vi "Start Sync.vi"(8 "error in (no error)":errorcluster, 11 "gRPC Server in":refnum<class "Query Server.lvclass">) -> (0 "error out":errorcluster, 3 "gRPC Server out":refnum<class "Query Server.lvclass">)   [LabVIEW 2019, in "Query Server.lvlib" / "Query Server.lvclass"]
uses:
  Query Server.lvclass
  gRPC lvSupport/Server API/typeDefs/grpcId.ctl
  Query Server.lvclass/Query Server.ctl
  RPC Messages/ServerEvent/ServerEvent_Data.ctl
  RPC Messages/QueryResponse/QueryResponse_Data.ctl
  RPC Messages/InvokeResponse/InvokeResponse_Data.ctl
  gRPC lvSupport/gprc-lvsupport.lvlib
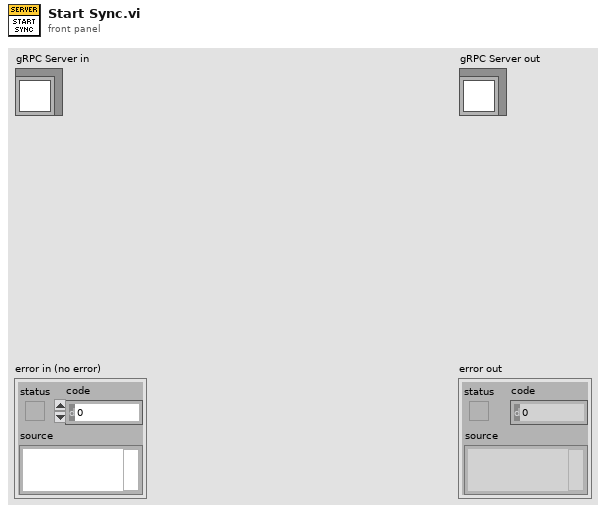
[diagram p1: front panel]
types:
  T1 = typedef "Query Server.lvlib/gprc-lvsupport.lvlib/grpcId.ctl" = u64
  T2 = typedef "Query Server.lvlib/Query Server.lvclass/ServerEvent_Data.ctl" = cluster{"eventData":string, "serverId":i32, "status":i32}
  T3 = typedef "Query Server.lvlib/Query Server.lvclass/QueryResponse_Data.ctl" = cluster{"message":string, "status":i32}
  T4 = typedef "Query Server.lvlib/Query Server.lvclass/InvokeResponse_Data.ctl" = cluster{"status":i32}
  T5 = typedef "Query Server.lvlib/Query Server.lvclass/Server gRPC UEs.ctl" = cluster{"Invoke gRPC UE":refnum<user-event>, "Query gRPC UE":refnum<user-event>, "Register gRPC UE":refnum<user-event>}
  T6 = typedef "Query Server.lvlib/Query Server.lvclass/RegistrationRequest_Data.ctl" = cluster{"eventName":string}
  T7 = typedef "Query Server.lvlib/Query Server.lvclass/QueryRequest_Data.ctl" = cluster{"query":string}
  T8 = typedef "Query Server.lvlib/Query Server.lvclass/InvokeRequest_Data.ctl" = cluster{"command":string, "parameter":string}
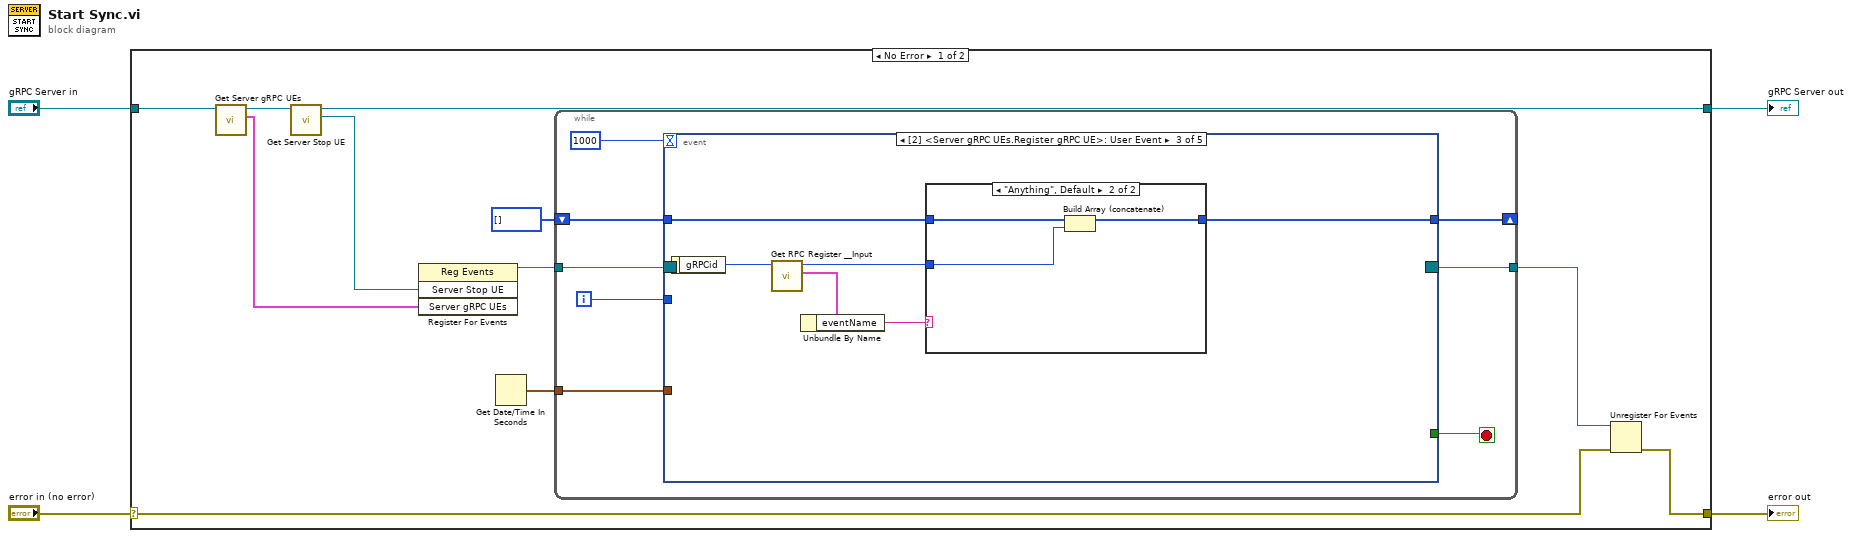
[diagram p0: block diagram]
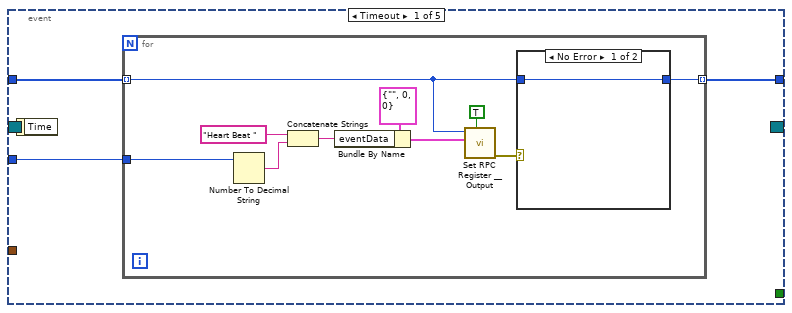
[diagram p2: hidden frame]
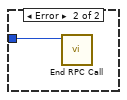
[diagram p3: hidden frame]
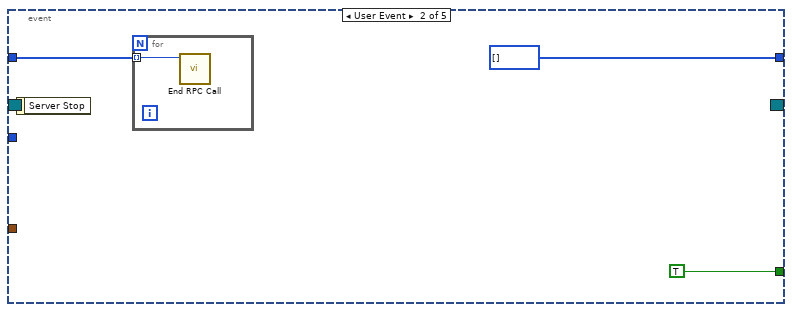
[diagram p4: hidden frame]
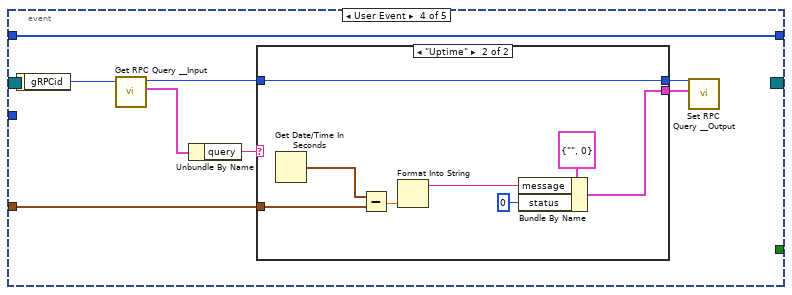
[diagram p6: hidden frame]
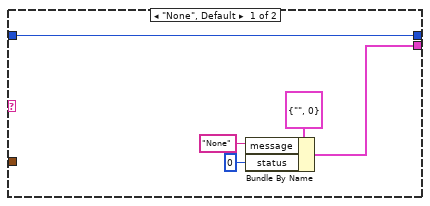
[diagram p7: hidden frame]
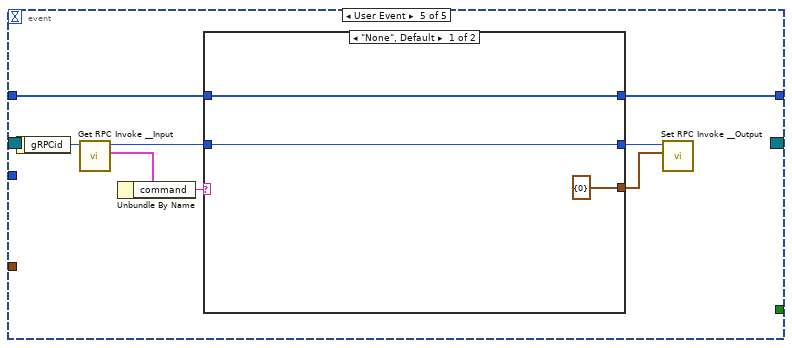
[diagram p8: hidden frame]
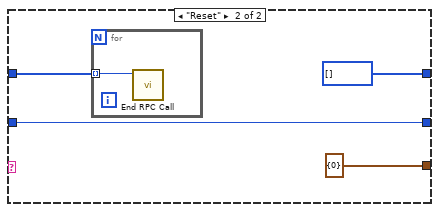
[diagram p9: hidden frame]
diagram:
  n1 = case shown="No Error" "error in (no error)" {
    selector: "error in (no error)" -> [w8 w91]
    tunnel: [w7 w91] -> w3
    tunnel: [w11 w90] -> w1
    tunnel: "gRPC Server in" -> [w15 w90]
    frame No Error {
      n2 = call "Get Server gRPC UEs.vi"("OOP Server in"=w15) -> ("Server gRPC UEs"=w12:T5, "OOP Server out"=w14:refnum<class "Query Server.lvclass">)  [unwired: 9 in]
      n3 = call "Get Server Stop UE.vi"("OOP Server in"=w14) -> ("Server Stop UE"=w13:refnum<user-event>, "OOP Server out"=w11:refnum<class "Query Server.lvclass">)  [unwired: 9 in]
      n4 = register-events(w13, w12) -> (reference out=w10:refnum<event-registration>)  [unwired: 2 in, 1 out]
      n5 = Get Date/Time In Seconds() -> (seconds since 1Jan1904=w6:timestamp)
      n6 = while {
        tunnel: w10 -> [w23]
        tunnel: [w21] -> w9
        shift-right: [w19] -> _
        shift-left: T1[] [] -> [w18]
        tunnel: w6 -> [w16]
        i -> [w17]
        stop <- w22 stop-if-true
        n7 = event "RPC Methods Event Structure" shown="[2] <Server gRPC UEs.Register gRPC UE>: User Event" {
          selector: w23 -> [_ _ _ _ _]
          dyn-events: [_ _ _ _ _] -> w21
          timeout: 1000 -> [_ _ _ _ _]
          tunnel: [_ TRUE _ _ _] -> w22
          tunnel: [w24 T1[] [] w44 w60 w74] -> w19
          tunnel: w18 -> [w26 w40 w43 w60 w81]
          tunnel: w17 -> [w25 _ _ _ _]
          tunnel: w16 -> [_ _ _ w54 _]
          event Timeout {
            n8 = event-data() -> ()  [unwired: 1 in, 1 out]
            n9 = for {
              tunnel: w26 -> [w30] mode=indexing
              tunnel: w25 -> [w31]
              tunnel: [w28] -> w24 mode=indexing
              n10 = Number To Decimal String(number=w31) -> (decimal integer string=w36:string)  [unwired: 1 in]
              n11 = Concatenate Strings("Heart Beat " ("eventdata"), w36) -> (w34:string)
              n12 = Bundle By Name(cluster=T2 {"eventData"="", "serverId"=0, "status"=0} ("Message Data"), "eventData"=w34) -> (w32:T2)
              n13 = call "Set RPC Register __Output.vi"("Streeming? (F)"=TRUE, "Message Data"=w32, "gRPCid in"=w30) -> ("error out"=w29:errorcluster)  [unwired: 8 in]
              n14 = case shown="No Error" w29 {
                tunnel: w30 -> [w37 w38]
                tunnel: [w37 _] -> w28
                frame No Error {
                }
                frame Error {
                  n15 = call "End RPC Call.vi"("gRPCid"=w38) -> ()  [unwired: 10 in, 1 out]
                }
              }
            }
          }
          event User Event {
            n16 = event-data() -> ()  [unwired: 1 in, 1 out]
            n17 = for {
              tunnel: w40 -> [w42] mode=indexing
              n18 = call "End RPC Call.vi"("gRPCid"=w42) -> ()  [unwired: 10 in, 1 out]
            }
          }
          event User Event {
            n19 = event-data() -> ("gRPCid"=w48:T1)  [unwired: 1 in]
            n20 = call "Get RPC Register __Input.vi"("gRPCid in"=w48) -> ("Message Data"=w47:T6, "gRPCid out"=w45:T1)  [unwired: 8 in, 1 out]
            n21 = Unbundle By Name(w47) -> ("eventName"=w46:string)
            n22 = case shown="\"Anything\", Default" w46 {
              tunnel: w45 -> [_ w52]
              tunnel: [w49 w51] -> w44
              tunnel: w43 -> [w49 w50]
              frame "None" {
              }
              frame "Anything", Default {
                n23 = Build Array (concatenate)(w50, w52) -> (w51:T1[])
              }
            }
          }
          event User Event {
            n24 = event-data() -> ("gRPCid"=w59:T1)  [unwired: 1 in]
            n25 = call "Get RPC Query __Input.vi"("gRPCid in"=w59) -> ("Message Data"=w58:T7, "gRPCid out"=w56:T1)  [unwired: 8 in, 1 out]
            n26 = Unbundle By Name(w58) -> ("query"=w57:string)
            n27 = case shown="\"Uptime\"" w57 {
              tunnel: w56 -> [w65 w73]
              tunnel: [w65 w73] -> w55
              tunnel: w54 -> [_ w68]
              tunnel: [w62 w66] -> w53
              frame "None", Default {
                n28 = Bundle By Name(cluster=T3 {"message"="", "status"=0} ("Message Data"), "message"="None", "status"=0) -> (w62:T3)
              }
              frame "Uptime" {
                n29 = Get Date/Time In Seconds() -> (seconds since 1Jan1904=w72:timestamp)
                n30 = Subtract(x=w72, y=w68) -> (x-y=w71:dbl)
                n31 = Format Into String(w71) -> (resulting string=w70:string)  [unwired: 3 in, 1 out]
                n32 = Bundle By Name(cluster=T3 {"message"="", "status"=0} ("Message Data"), "message"=w70, "status"=0) -> (w66:T3)
              }
            }
            n33 = call "Set RPC Query __Output.vi"("Message Data"=w53, "gRPCid in"=w55) -> ()  [unwired: 9 in, 1 out]
          }
          event User Event {
            n34 = event-data() -> ("gRPCid"=w80:T1)  [unwired: 1 in]
            n35 = call "Get RPC Invoke __Input.vi"("gRPCid in"=w80) -> ("Message Data"=w79:T8, "gRPCid out"=w77:T1)  [unwired: 8 in, 1 out]
            n36 = Unbundle By Name(w79) -> ("command"=w78:string)
            n37 = case shown="\"None\", Default" w78 {
              tunnel: w81 -> [w84 w86]
              tunnel: w77 -> [w83 w88]
              tunnel: [w83 w88] -> w76
              tunnel: [T4 {"status"=0} ("Message Data") T4 {"status"=0} ("Message Data")] -> w75
              tunnel: [w84 T1[] []] -> w74
              frame "None", Default {
              }
              frame "Reset" {
                n38 = for {
                  tunnel: w86 -> [w89] mode=indexing
                  n39 = call "End RPC Call.vi"("gRPCid"=w89) -> ()  [unwired: 10 in, 1 out]
                }
              }
            }
            n40 = call "Set RPC Invoke __Output.vi"("Message Data"=w75, "gRPCid in"=w76) -> ()  [unwired: 9 in, 1 out]
          }
        }
      }
      n41 = Unregister For Events(event registration refnum=w9, error in=w8) -> (error out=w7:errorcluster)
    }
    frame Error {
    }
  }
  "error out" <- w3
  "gRPC Server out" <- w1
